vi "write_attributes.vi"(8 "error in (no error)":errorcluster, 10 "attributes":T1, 11 "RadiusNeighborsRegressor in":refnum<class "RadiusNeighborsRegressor.lvclass">) -> (0 "error out":errorcluster, 3 "RadiusNeighborsRegressor out":refnum<class "RadiusNeighborsRegressor.lvclass">)   [LabVIEW 2020, in "RadiusNeighborsRegressor.lvclass"]
uses:
  RadiusNeighborsRegressor.lvclass
  Controls/radius_neighbors_regressor_attributes.ctl
  RadiusNeighborsRegressor.lvclass/RadiusNeighborsRegressor.ctl
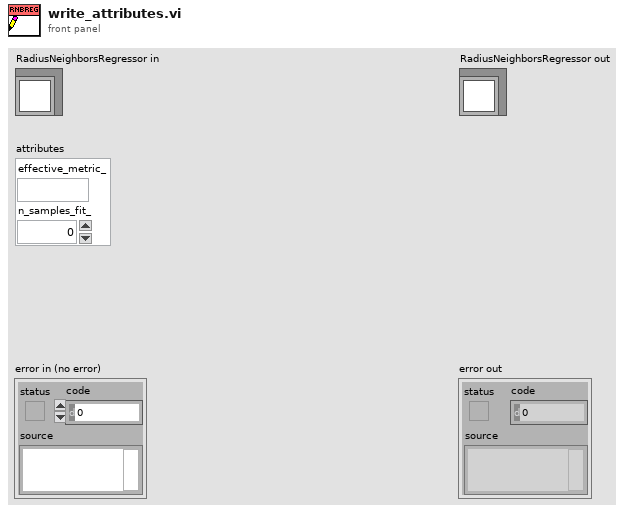
[diagram p1: front panel]
types:
  T1 = typedef "radius_neighbors_regressor_attributes.ctl" = cluster{"effective_metric_":string, "n_samples_fit_":dbl}
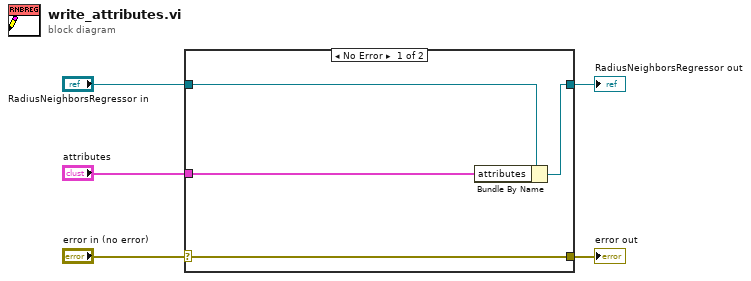
[diagram p0: block diagram]
diagram:
  n1 = case shown="No Error" "error in (no error)" {
    selector: "error in (no error)" -> [w9 w10]
    tunnel: [w9 w10] -> w4
    tunnel: [w7 w11] -> w2
    tunnel: "RadiusNeighborsRegressor in" -> [w8 w11]
    tunnel: "attributes" -> [w6 _]
    frame No Error {
      n2 = Bundle By Name(cluster=w8, "attributes"=w6) -> (w7:refnum<class "RadiusNeighborsRegressor.lvclass">)
    }
    frame Error {
    }
  }
  "error out" <- w4
  "RadiusNeighborsRegressor out" <- w2
